vi "svx_Colormap Exec Commands.vi"(5 "Container ref":refnum<vi>, 6 "This VI":refnum<vi>, 7 "Colormap ref":refnum<vi>, 9 "Events":T2[](array[typedef])=[enum."[Data] Update"], 10 "State in":T1={"RefQueue"=refnum, "Properties/Undo"=refnum, "Bound"={"Width"=0, "Height"=0}, "Plot Area:Colors"={"FG Color"=11776947, "BG Color"=0}, "scale legend visible?"=FALSE, "graph palette visible?"=FALSE, "cursor palette visible?"=FALSE, "Ignore Array"=TRUE, "Smooth Update"=FALSE, "Z Scale"={"Z Scale.Scale Fit"=2, "Z Scale.Name Label.Text"="Amplitude", "Z Scale.Interpolate Color"=TRUE, "Visible"=TRUE, "Label Visible"=TRUE, "format string"="%#.2g", "Z Scale.Range"={"Minimum"=0.0, "Maximum"=500.0}}, "X Scale"={"X Scale.Scale Fit"=2, "X Scale.Offset and Multiplier"={"Offset"=0.0, "Multiplier"=1.0}, "X Scale.Name Label.Text"="Time", "X Scale.Range"={"Minimum"=0.0, "Maximum"=10.0}, "Visible"=TRUE, "Label Visible"=TRUE, "format string"="%#.2g"}, "Y Scale"={"Y Scale.Scale Fit"=2, "Y Scale.Offset and Multiplier"={"Offset"=0.0, "Multiplier"=1.0}, "Y Scale.Name Label.Text"="Frequency", "Y Scale.Range"={"Minimum"=0.0, "Maximum"=500.0}, "Visible"=TRUE, "Label Visible"=TRUE, "format string"="%#.2g"}, "Annotation List"=[], "Cursor List"=[], "Display Frequency Lines"=TRUE, "Display Order Lines"=TRUE, "Display Order text"=TRUE, "Display Frequency text"=TRUE, "Order Lineproperty"={"Line"={"Width"=1, "Style"=enum."Dash"}, "color"=0}, "Order Textproperty"={"Test size"=11, "color"=16777222, "background"=16777216}, "Orders"=[], "Frequency"=[], "Frequency Lineproperty"={"Line"={"Width"=1, "Style"=enum."Dash"}, "color"=0}, "Frequency Textproperty"={"Test size"=11, "color"=16777222, "background"=16777216}, "Display Order from Cursor"=FALSE, "Display Freq from Cursor"=FALSE, "Active Cursor"=0, "Selected Cursors"=[], "Cursor Move"=refnum, "Scale Range Change"=refnum}, 11 "Data in":T3 {"Y scale"."multiplier" format="%.2f"; "Y scale"."offset" format="%.2f"; "X scale"."multiplier" format="%.2f"; "X scale"."offset" format="%.2f"; "spectral map" format="%.2f"}) -> (2 "State out":T1={"RefQueue"=refnum, "Properties/Undo"=refnum, "Bound"={"Width"=0, "Height"=0}, "Plot Area:Colors"={"FG Color"=11776947, "BG Color"=0}, "scale legend visible?"=FALSE, "graph palette visible?"=FALSE, "cursor palette visible?"=FALSE, "Ignore Array"=TRUE, "Smooth Update"=FALSE, "Z Scale"={"Z Scale.Scale Fit"=2, "Z Scale.Name Label.Text"="Amplitude", "Z Scale.Interpolate Color"=TRUE, "Visible"=TRUE, "Label Visible"=TRUE, "format string"="%#.2g", "Z Scale.Range"={"Minimum"=0.0, "Maximum"=500.0}}, "X Scale"={"X Scale.Scale Fit"=2, "X Scale.Offset and Multiplier"={"Offset"=0.0, "Multiplier"=1.0}, "X Scale.Name Label.Text"="Time", "X Scale.Range"={"Minimum"=0.0, "Maximum"=10.0}, "Visible"=TRUE, "Label Visible"=TRUE, "format string"="%#.2g"}, "Y Scale"={"Y Scale.Scale Fit"=2, "Y Scale.Offset and Multiplier"={"Offset"=0.0, "Multiplier"=1.0}, "Y Scale.Name Label.Text"="Frequency", "Y Scale.Range"={"Minimum"=0.0, "Maximum"=500.0}, "Visible"=TRUE, "Label Visible"=TRUE, "format string"="%#.2g"}, "Annotation List"=[], "Cursor List"=[], "Display Frequency Lines"=TRUE, "Display Order Lines"=TRUE, "Display Order text"=TRUE, "Display Frequency text"=TRUE, "Order Lineproperty"={"Line"={"Width"=1, "Style"=enum."Dash"}, "color"=0}, "Order Textproperty"={"Test size"=11, "color"=16777222, "background"=16777216}, "Orders"=[], "Frequency"=[], "Frequency Lineproperty"={"Line"={"Width"=1, "Style"=enum."Dash"}, "color"=0}, "Frequency Textproperty"={"Test size"=11, "color"=16777222, "background"=16777216}, "Display Order from Cursor"=FALSE, "Display Freq from Cursor"=FALSE, "Active Cursor"=0, "Selected Cursors"=[], "Cursor Move"=refnum, "Scale Range Change"=refnum})   [LabVIEW 2017, in "SVX Colormap.xctl"]
uses:
  <vilib>/addons/_XControls/Colormap/SVX Colormap.xctl
  <vilib>/addons/_XControls/Colormap/subVIs/svx_Colormap Data.ctl
  <vilib>/addons/_XControls/Colormap/TypeDef/svx_Colormap_Event.ctl
  <vilib>/addons/_XControls/Colormap/subVIs/svx_Colormap State.ctl
  <vilib>/addons/_XControls/Colormap/TypeDef/svx_Colormap_InnerState.ctl
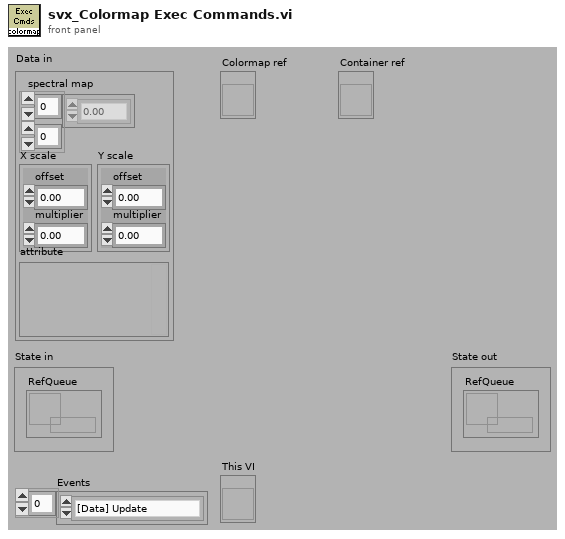
[diagram p1: front panel]
types:
  T1 = typedef "SVX Colormap.xctl/svx_Colormap State.ctl" = cluster{"RefQueue":refnum<queue>, "Properties/Undo":refnum<queue>, "Bound":cluster{"Width":u32, "Height":u32}, "Plot Area:Colors":cluster{"FG Color":u32, "BG Color":u32}, "scale legend visible?":bool, "graph palette visible?":bool, "cursor palette visible?":bool, "Ignore Array":bool, "Smooth Update":bool, "Z Scale":cluster{"Z Scale.Scale Fit":u8, "Z Scale.Name Label.Text":string, "Z Scale.Interpolate Color":bool, "Visible":bool, "Label Visible":bool, "format string":string, "Z Scale.Range":cluster{"Minimum":dbl, "Maximum":dbl}}, "X Scale":cluster{"X Scale.Scale Fit":u8, "X Scale.Offset and Multiplier":cluster{"Offset":dbl, "Multiplier":dbl}, "X Scale.Name Label.Text":string, "X Scale.Range":cluster{"Minimum":dbl, "Maximum":dbl}, "Visible":bool, "Label Visible":bool, "format string":string}, "Y Scale":cluster{"Y Scale.Scale Fit":u8, "Y Scale.Offset and Multiplier":cluster{"Offset":dbl, "Multiplier":dbl}, "Y Scale.Name Label.Text":string, "Y Scale.Range":cluster{"Minimum":dbl, "Maximum":dbl}, "Visible":bool, "Label Visible":bool, "format string":string}, "Annotation List":cluster{"Name":string, "Color":u32, "Style":u8, "Point Style":u8, "Name Visible":bool, "Allow Drag":bool, "Annotation Mode":u32, "Plot":i32, "Index":i32, "Position":cluster{"X":dbl, "Y":dbl}, "X Scale":u32, "Y Scale":u32, "Show Arrow":bool, "Lock Name":bool, "Plot Area":i32, "Label Offset":cluster{"X":dbl, "Y":dbl}}[], "Cursor List":cluster{"Name":string, "Color":u32, "Style":u8, "Point Style":u8, "Name Visible":bool, "Allow Drag":bool, "Cursor Mode":u32, "Plot":i32, "Index":i32, "Position":cluster{"X":dbl, "Y":dbl}, "X Scale":u32, "Y Scale":u32, "Watch Plots":i32[], "Watch All Plots":bool, "Plot Area":i32, "Label Offset":cluster{"X":dbl, "Y":dbl}}[], "Display Frequency Lines":bool, "Display Order Lines":bool, "Display Order text":bool, "Display Frequency text":bool, "Order Lineproperty":cluster{"Line":cluster{"Width":u16, "Style":enum32{"Solid", "Dash", "Dot", "DashDot", "DashDotDot"}}, "color":u32}, "Order Textproperty":cluster{"Test size":i16, "color":u32, "background":u32}, "Orders":dbl[], "Frequency":dbl[], "Frequency Lineproperty":cluster{"Line":cluster{"Width":u16, "Style":enum32{"Solid", "Dash", "Dot", "DashDot", "DashDotDot"}}, "color":u32}, "Frequency Textproperty":cluster{"Test size":i16, "color":u32, "background":u32}, "Display Order from Cursor":bool, "Display Freq from Cursor":bool, "Active Cursor":u32, "Selected Cursors":u32[], "Cursor Move":refnum<user-event>, "Scale Range Change":refnum<user-event>}
  T2 = typedef "SVX Colormap.xctl/svx_Colormap_Event.ctl" = enum16{"None", "[Axis] X Range", "[Axis] Y Range", "[Axis] Z Range", "[Axis] Range", "[Axis] X FString", "[Axis] Y FString", "[Axis] Z FString", "[Axis] X Name", "[Axis] X ScaleVis", "[Axis] X NameVis", "[Axis] Y Name", "[Axis] Y ScaleVis", "[Axis] Y NameVis", "[Axis] Z Name", "[Axis] Z ScaleVis", "[Axis] Z NameVis", "[Image] Line", "[Axis] Z Interp", "[Data] Update", "[Layout] Resize", "[ColorTable] Ignore Array", "[Legend] ScaleVis", "[Legend] GPVis", "[Legend] CPVis", "[Smooth] Update", "[Cursor] Update", "[Plot Area] Colors", "[Size] Minimum", "[Annotation] Update", "[Properties Dialog]", "[Axis] Autoscale X", "[Axis] Autoscale Y", "[Axis] Autoscale Z"}
  T3 = typedef "SVX Colormap.xctl/svx_Colormap Data.ctl" = cluster{"spectral map":dbl[][], "X scale":cluster{"offset":dbl, "multiplier":dbl}, "Y scale":cluster{"offset":dbl, "multiplier":dbl}, "attribute":variant}
  T4 = cluster{"Name":string, "Color":u32, "Style":u8, "Point Style":u8, "Name Visible":bool, "Allow Drag":bool, "Cursor Mode":u32, "Plot":i32, "Index":i32, "Position":cluster{"X":dbl, "Y":dbl}, "X Scale":u32, "Y Scale":u32, "Watch Plots":i32[], "Watch All Plots":bool, "Plot Area":i32, "Label Offset":cluster{"X":dbl, "Y":dbl}}[]
  T5 = cluster{"Name":string, "Color":u32, "Style":u8, "Point Style":u8, "Name Visible":bool, "Allow Drag":bool, "Annotation Mode":u32, "Plot":i32, "Index":i32, "Position":cluster{"X":dbl, "Y":dbl}, "X Scale":u32, "Y Scale":u32, "Show Arrow":bool, "Lock Name":bool, "Plot Area":i32, "Label Offset":cluster{"X":dbl, "Y":dbl}}[]
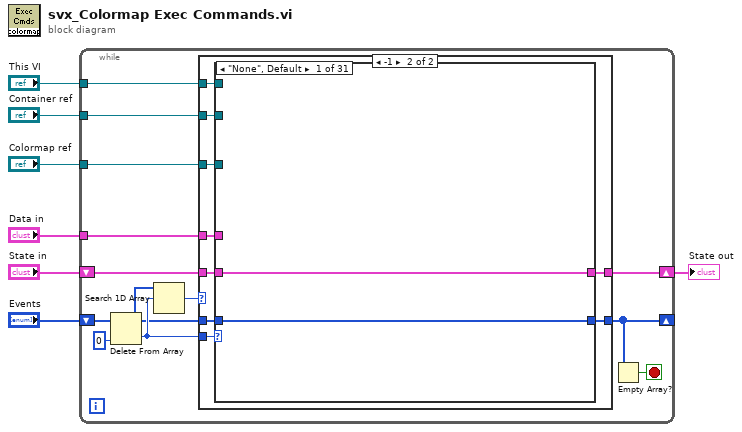
[diagram p0: block diagram]
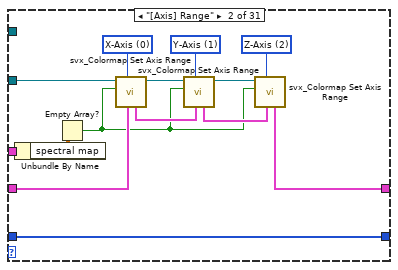
[diagram p3: hidden frame]
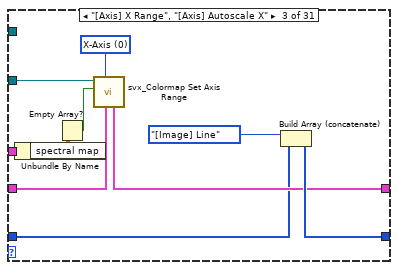
[diagram p4: hidden frame]
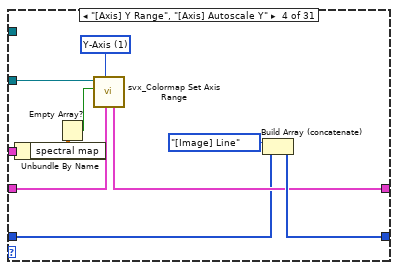
[diagram p5: hidden frame]
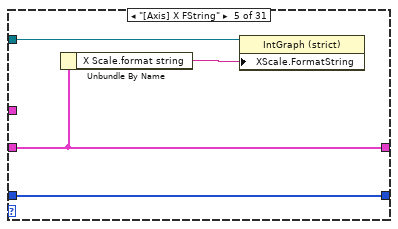
[diagram p6: hidden frame]
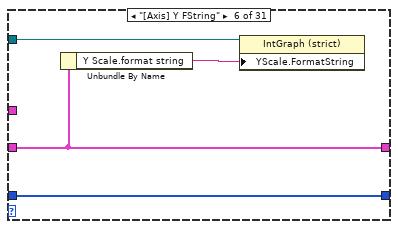
[diagram p7: hidden frame]
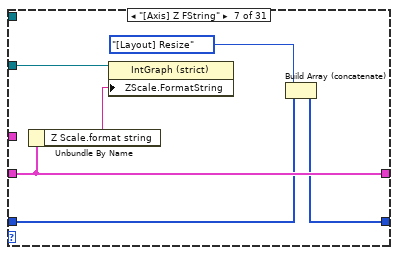
[diagram p8: hidden frame]
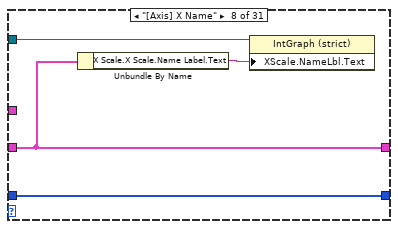
[diagram p9: hidden frame]
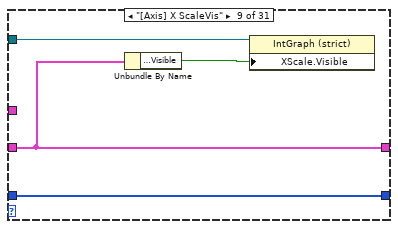
[diagram p10: hidden frame]
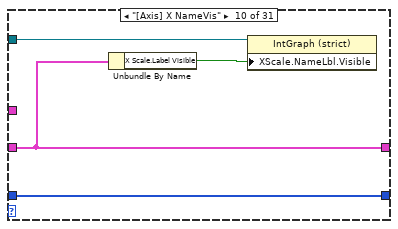
[diagram p11: hidden frame]
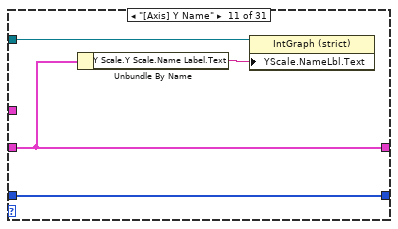
[diagram p12: hidden frame]
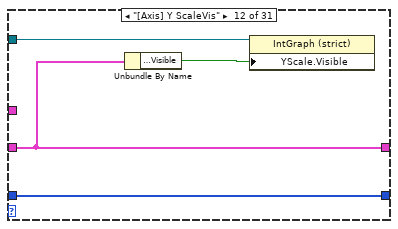
[diagram p13: hidden frame]
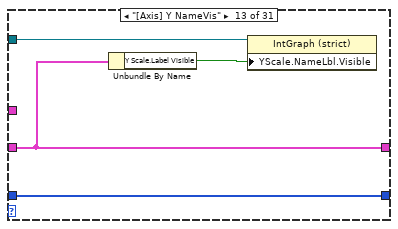
[diagram p14: hidden frame]
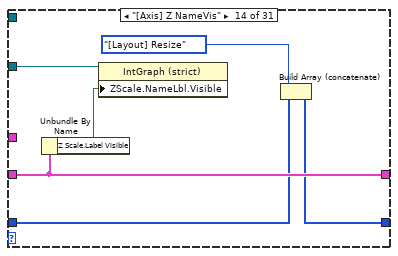
[diagram p15: hidden frame]
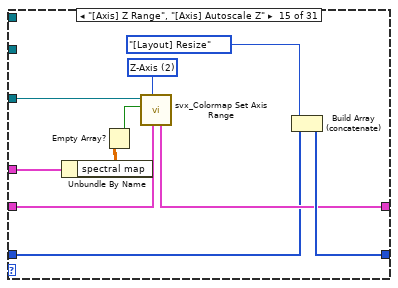
[diagram p16: hidden frame]
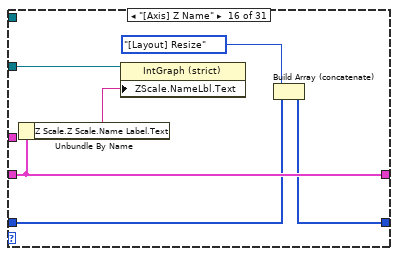
[diagram p17: hidden frame]
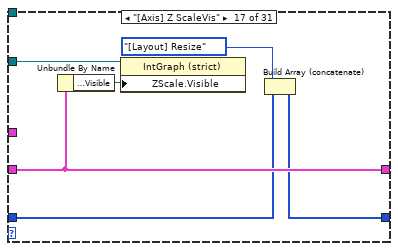
[diagram p18: hidden frame]
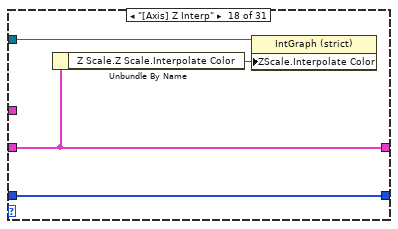
[diagram p19: hidden frame]
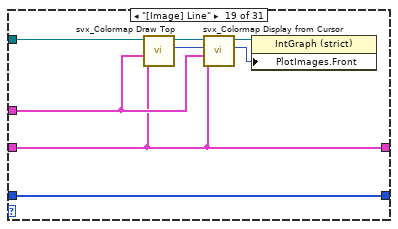
[diagram p20: hidden frame]
diagram:
  n1 = while {
    tunnel: "Data in" -> [w20]
    tunnel: "Colormap ref" -> [w19]
    shift-right: [w13] -> w1
    shift-left: "State in" -> [w18]
    shift-right: [w15] -> _
    shift-left: "Events" -> [w16]
    tunnel: "Container ref" -> [w12]
    tunnel: "This VI" -> [w8]
    stop <- w14 stop-if-true
    n2 = Delete From Array(array=w16, index=0) -> (deleted portion=w11:T2, array with subset deleted=w10:T2[])  [unwired: 1 in]
    n3 = Search 1D Array(1D array=w10, element=w11) -> (index of element=w9:i32)  [unwired: 1 in]
    n4 = case shown="-1" w9 {
      tunnel: w20 -> [_ w31]
      tunnel: w19 -> [_ w30]
      tunnel: w18 -> [w22 w29]
      tunnel: [w21 w28] -> w15
      tunnel: [w22 w27] -> w13
      tunnel: w12 -> [_ w26]
      tunnel: w11 -> [_ w25]
      tunnel: w10 -> [w21 w24]
      tunnel: w8 -> [_ w23]
      frame Default {
      }
      frame -1 {
        n5 = case shown="\"None\", Default" w25 {
          tunnel: w31 -> [_ w45 w55 w65 _ _ _ _ _ _ _ _ _ _ w116 _ _ _ w144 _ w155 _ _ _ _ _ _ _ _ _ _]
          tunnel: w29 -> [w33 w43 w53 w63 w69 w73 w80 w84 w88 w92 w96 w100 w104 w111 w115 w126 w133 w135 w138 w147 w154 w162 w172 w178 w185 w189 w202 w206 w213 w218 w223]
          tunnel: w30 -> [_ w46 w56 w66 w71 w75 w78 w85 w89 w93 w97 w101 w105 w108 w118 w124 w130 w137 w145 w148 w156 w167 w174 w180 w187 w191 w204 w208 _ w221 _]
          tunnel: w24 -> [w32 w34 w48 w59 w68 w72 w77 w83 w87 w91 w95 w99 w103 w106 w113 w122 w128 w134 w143 w146 w152 w161 w169 w175 w182 w188 w199 w205 w212 w219 _]
          tunnel: [w32 w34 w51 w61 w68 w72 w79 w83 w87 w91 w95 w99 w103 w110 w121 w125 w132 w134 w143 w146 w151 w161 w171 w177 w184 w188 w198 w205 w212 w219 w222] -> w28
          tunnel: [w33 w35 w50 w60 w69 w73 w80 w84 w88 w92 w96 w100 w104 w111 w114 w126 w133 w135 w138 w147 w153 w162 w172 w178 w185 w189 w202 w206 w213 w218 w223] -> w27
          tunnel: w26 -> [_ _ _ _ _ _ _ _ _ _ _ _ _ _ _ _ _ _ _ w149 _ _ _ _ _ _ _ _ _ _ _]
          tunnel: w23 -> [_ _ _ _ _ _ _ _ _ _ _ _ _ _ _ _ _ _ _ _ _ _ _ _ _ _ _ _ w214 _ _]
          frame "None", Default {
          }
          frame "[Axis] Range" {
            w41 = u16 2 items=["X-Axis", "Y-Axis", "Z-Axis"] ("axis selection")
            w42 = u16 1 items=["X-Axis", "Y-Axis", "Z-Axis"] ("axis selection")
            w47 = u16 0 items=["X-Axis", "Y-Axis", "Z-Axis"] ("axis selection")
            n6 = Unbundle By Name(w45) -> ("spectral map"=w44:dbl[][])
            n7 = Empty Array?(array=w44) -> (empty?=w36:bool)
            n8 = call <vilib>:"svx_Colormap Set Axis Range.vi"("State in"=w43, "axis selection"=w47, "empty?"=w36, "Color Map in"=w46) -> ("Color Map out"=w39:refnum<vi>, "State out"=w40:T1)  [unwired: 5 in, 1 out]
            n9 = call <vilib>:"svx_Colormap Set Axis Range.vi"("State in"=w40, "axis selection"=w42, "empty?"=w36, "Color Map in"=w39) -> ("Color Map out"=w37:refnum<vi>, "State out"=w38:T1)  [unwired: 5 in, 1 out]
            n10 = call <vilib>:"svx_Colormap Set Axis Range.vi"("State in"=w38, "axis selection"=w41, "empty?"=w36, "Color Map in"=w37) -> ("State out"=w35:T1)  [unwired: 5 in, 2 out]
          }
          frame "[Axis] X Range", "[Axis] Autoscale X" {
            w57 = u16 0 items=["X-Axis", "Y-Axis", "Z-Axis"] ("axis selection")
            n11 = Unbundle By Name(w55) -> ("spectral map"=w54:dbl[][])
            n12 = Empty Array?(array=w54) -> (empty?=w52:bool)
            n13 = call <vilib>:"svx_Colormap Set Axis Range.vi"("State in"=w53, "axis selection"=w57, "empty?"=w52, "Color Map in"=w56) -> ("State out"=w50:T1)  [unwired: 5 in, 2 out]
            n14 = Build Array (concatenate)(svx_Colormap_Event."[Image] Line" ("Property Page User Events"), w48) -> (w51:T2[])
          }
          frame "[Axis] Y Range", "[Axis] Autoscale Y" {
            w67 = u16 1 items=["X-Axis", "Y-Axis", "Z-Axis"] ("axis selection")
            n15 = Unbundle By Name(w65) -> ("spectral map"=w64:dbl[][])
            n16 = Empty Array?(array=w64) -> (empty?=w62:bool)
            n17 = call <vilib>:"svx_Colormap Set Axis Range.vi"("State in"=w63, "axis selection"=w67, "empty?"=w62, "Color Map in"=w66) -> ("State out"=w60:T1)  [unwired: 5 in, 2 out]
            n18 = Build Array (concatenate)(svx_Colormap_Event."[Image] Line" ("Property Page User Events"), w59) -> (w61:T2[])
          }
          frame "[Axis] X FString" {
            n19 = Unbundle By Name(w69) -> ("X Scale.format string"=w70:string)
            n20 = property class="IntGraph (strict)"(reference=w71, "XScale.FormatString"=w70) -> ()  [unwired: 1 in, 2 out]
          }
          frame "[Axis] Y FString" {
            n21 = Unbundle By Name(w73) -> ("Y Scale.format string"=w74:string)
            n22 = property class="IntGraph (strict)"(reference=w75, "YScale.FormatString"=w74) -> ()  [unwired: 1 in, 2 out]
          }
          frame "[Axis] Z FString" {
            n23 = Unbundle By Name(w80) -> ("Z Scale.format string"=w81:string)
            n24 = property class="IntGraph (strict)"(reference=w78, "ZScale.FormatString"=w81) -> ()  [unwired: 1 in, 2 out]
            n25 = Build Array (concatenate)(svx_Colormap_Event."[Layout] Resize" ("Property Page User Events"), w77) -> (w79:T2[])
          }
          frame "[Axis] X Name" {
            n26 = Unbundle By Name(w84) -> ("X Scale.X Scale.Name Label.Text"=w82:string)
            n27 = property class="IntGraph (strict)"(reference=w85, "XScale.NameLbl.Text"=w82) -> ()  [unwired: 1 in, 2 out]
          }
          frame "[Axis] X ScaleVis" {
            n28 = Unbundle By Name(w88) -> ("X Scale.Visible"=w86:bool)
            n29 = property class="IntGraph (strict)"(reference=w89, "XScale.Visible"=w86) -> ()  [unwired: 1 in, 2 out]
          }
          frame "[Axis] X NameVis" {
            n30 = Unbundle By Name(w92) -> ("X Scale.Label Visible"=w90:bool)
            n31 = property class="IntGraph (strict)"(reference=w93, "XScale.NameLbl.Visible"=w90) -> ()  [unwired: 1 in, 2 out]
          }
          frame "[Axis] Y Name" {
            n32 = Unbundle By Name(w96) -> ("Y Scale.Y Scale.Name Label.Text"=w94:string)
            n33 = property class="IntGraph (strict)"(reference=w97, "YScale.NameLbl.Text"=w94) -> ()  [unwired: 1 in, 2 out]
          }
          frame "[Axis] Y ScaleVis" {
            n34 = Unbundle By Name(w100) -> ("Y Scale.Visible"=w98:bool)
            n35 = property class="IntGraph (strict)"(reference=w101, "YScale.Visible"=w98) -> ()  [unwired: 1 in, 2 out]
          }
          frame "[Axis] Y NameVis" {
            n36 = Unbundle By Name(w104) -> ("Y Scale.Label Visible"=w102:bool)
            n37 = property class="IntGraph (strict)"(reference=w105, "YScale.NameLbl.Visible"=w102) -> ()  [unwired: 1 in, 2 out]
          }
          frame "[Axis] Z NameVis" {
            n38 = Unbundle By Name(w111) -> ("Z Scale.Label Visible"=w109:bool)
            n39 = property class="IntGraph (strict)"(reference=w108, "ZScale.NameLbl.Visible"=w109) -> ()  [unwired: 1 in, 2 out]
            n40 = Build Array (concatenate)(svx_Colormap_Event."[Layout] Resize" ("Property Page User Events"), w106) -> (w110:T2[])
          }
          frame "[Axis] Z Range", "[Axis] Autoscale Z" {
            w117 = u16 2 items=["X-Axis", "Y-Axis", "Z-Axis"] ("axis selection")
            n41 = Unbundle By Name(w116) -> ("spectral map"=w120:dbl[][])
            n42 = Empty Array?(array=w120) -> (empty?=w119:bool)
            n43 = call <vilib>:"svx_Colormap Set Axis Range.vi"("State in"=w115, "axis selection"=w117, "empty?"=w119, "Color Map in"=w118) -> ("State out"=w114:T1)  [unwired: 5 in, 2 out]
            n44 = Build Array (concatenate)(svx_Colormap_Event."[Layout] Resize" ("Property Page User Events"), w113) -> (w121:T2[])
          }
          frame "[Axis] Z Name" {
            n45 = Unbundle By Name(w126) -> ("Z Scale.Z Scale.Name Label.Text"=w127:string)
            n46 = property class="IntGraph (strict)"(reference=w124, "ZScale.NameLbl.Text"=w127) -> ()  [unwired: 1 in, 2 out]
            n47 = Build Array (concatenate)(svx_Colormap_Event."[Layout] Resize" ("Property Page User Events"), w122) -> (w125:T2[])
          }
          frame "[Axis] Z ScaleVis" {
            n48 = Unbundle By Name(w133) -> ("Z Scale.Visible"=w131:bool)
            n49 = property class="IntGraph (strict)"(reference=w130, "ZScale.Visible"=w131) -> ()  [unwired: 1 in, 2 out]
            n50 = Build Array (concatenate)(svx_Colormap_Event."[Layout] Resize" ("Property Page User Events"), w128) -> (w132:T2[])
          }
          frame "[Axis] Z Interp" {
            n51 = Unbundle By Name(w135) -> ("Z Scale.Z Scale.Interpolate Color"=w136:bool)
            n52 = property class="IntGraph (strict)"(reference=w137, "ZScale.Interpolate Color"=w136) -> ()  [unwired: 1 in, 2 out]
          }
          frame "[Image] Line" {
            n53 = call <vilib>:"svx_Colormap Draw Top.vi"("State"=w138, "Data In"=w144, "Color Map in"=w145) -> ("new picture out"=w142:picture, "Color Map out"=w141:refnum<vi>)  [unwired: 7 in]
            n54 = call <vilib>:"svx_Colormap Display from Cursor.vi"("State"=w138, "Data In"=w144, "new picture in"=w142, "Color Map in"=w141) -> ("new picture out"=w139:picture, "Color Map out"=w140:refnum<vi>)  [unwired: 6 in]
            n55 = property class="IntGraph (strict)"(reference=w140, "PlotImages.Front"=w139) -> ()  [unwired: 1 in, 2 out]
          }
          frame "[Layout] Resize" {
            n56 = call <vilib>:"svx_Colormap Resize Pane for Scale and Cursor Legend.vi"("Color Map in"=w148, "Container ref"=w149) -> ()  [unwired: 10 in]
          }
          frame "[Data] Update" {
            w150 = T2[] [enum."[ColorTable] Ignore Array", enum."[Axis] Range", enum."[Image] Line"] items=["None", "[Axis] X Range", "[Axis] Y Range", "[Axis] Z Range", "[Axis] Range", "[Axis] X FString", "[Axis] Y FString", "[Axis] Z FString", "[Axis] X Name", "[Axis] X ScaleVis", "[Axis] X NameVis", "[Axis] Y Name", "[Axis] Y ScaleVis", "[Axis] Y NameVis", "[Axis] Z Name", "[Axis] Z ScaleVis", "[Axis] Z NameVis", "[Image] Line", "[Axis] Z Interp", "[Data] Update", "[Layout] Resize", "[ColorTable] Ignore Array", "[Legend] ScaleVis", "[Legend] GPVis", "[Legend] CPVis", "[Smooth] Update", "[Cursor] Update", "[Plot Area] Colors", "[Size] Minimum", "[Annotation] Update", "[Properties Dialog]", "[Axis] Autoscale X", "[Axis] Autoscale Y", "[Axis] Autoscale Z"]
            n57 = Unbundle By Name(w155) -> ("X scale"=w159:cluster{"offset":dbl, "multiplier":dbl}, "Y scale"=w158:cluster{"offset":dbl, "multiplier":dbl}, "spectral map"=w157:dbl[][])
            n58 = property class="IntGraph (strict)"(reference=w156, "XScale.Ofst&Mult"=w159, "YScale.Ofst&Mult"=w158, "Val(Sgnl)"=w157) -> ()  [unwired: 1 in, 2 out]
            n59 = Bundle By Name(cluster=w154, "X Scale.X Scale.Offset and Multiplier"=w159, "Y Scale.Y Scale.Offset and Multiplier"=w158) -> (w153:T1)
            n60 = Build Array (concatenate)(w150, w152) -> (w151:T2[])
          }
          frame "[ColorTable] Ignore Array" {
            w165 = u32[] [0, 0, 2, 4, 6, 8, 10, 12, 14, 16, 18, 20, 22, 24, 26, 28, 30, 32, 34, 36, 38, 40, 42, 44, 46, 48, 50, 52, 54, 56, 58, 60, 62, 64, 66, 68, 70, 72, 74, 76, 78, 80, 82, 84, 86, 88, 90, 92, 94, 96, 98, 100, 102, 104, 106, 108, 110, 112, 114, 116, 118, 120, 122, 124, 126, 128, 130, 132, 134, 136, 138, 140, 142, 144, 146, 148, 150, 152, 154, 156, 158, 160, 162, 164, 166, 168, 170, 172, 174, 176, 178, 180, 182, 184, 186, 188, 190, 192, 194, 196, 198, 200, 202, 204, 206, 208, 210, 212, 214, 216, 218, 220, 222, 224, 226, 228, 230, 232, 234, 236, 238, 240, 242, 244, 246, 248, 250, 252, 255, 131839, 263423, 395007, 526591, 658175, 789759, 921343, 1052927, 1184511, 1316095, 1447679, 1579263, 1710847, 1842431, 1974015, 2105599, 2237183, 2368767, 2500351, 2631935, 2763519, 2895103, 3026687, 3158271, 3289855, 3421439, 3553023, 3684607, 3816191, 3947775, 4079359, 4210943, 4342527, 4474111, 4605695, 4737279, 4868863, 5000447, 5132031, 5263615, 5395199, 5526783, 5658367, 5789951, 5921535, 6053119, 6184703, 6316287, 6447871, 6579455, 6711039, 6842623, 6974207, 7105791, 7237375, 7368959, 7500543, 7632127, 7763711, 7895295, 8026879, 8158463, 8290047, 8421631, 8553215, 8684799, 8816383, 8947967, 9079551, 9211135, 9342719, 9474303, 9605887, 9737471, 9869055, 10000639, 10132223, 10263807, 10395391, 10526975, 10658559, 10790143, 10921727, 11053311, 11184895, 11316479, 11448063, 11579647, 11711231, 11842815, 11974399, 12105983, 12237567, 12369151, 12500735, 12632319, 12763903, 12895487, 13027071, 13158655, 13290239, 13421823, 13553407, 13684991, 13816575, 13948159, 14079743, 14211327, 14342911, 14474495, 14606079, 14737663, 14869247, 15000831, 15132415, 15263999, 15395583, 15527167, 15658751, 15790335, 15921919, 16053503, 16185087, 16316671, 16448255, 16579839, 16777215]  # Color Table
            w166 = u32[] [0, 8388863, 8257791, 8061183, 7930111, 7733503, 7602431, 7405823, 7274751, 7078143, 6947071, 6750463, 6619391, 6422783, 6291711, 6095103, 5964031, 5767423, 5636351, 5439743, 5308671, 5112063, 4980991, 4784383, 4653311, 4456703, 4325631, 4129023, 3932415, 3801343, 3604735, 3473663, 3277055, 3145983, 2949375, 2818303, 2621695, 2490623, 2294015, 2162943, 1966335, 1835263, 1638655, 1507583, 1310975, 1179903, 983295, 852223, 655615, 524543, 327935, 196863, 511, 1791, 3071, 4351, 5631, 6911, 8191, 9471, 10751, 12031, 13311, 14591, 15871, 17151, 18431, 19711, 20991, 22271, 23551, 24831, 26111, 27391, 28671, 29951, 31231, 32511, 33791, 35071, 36351, 37631, 38911, 40191, 41471, 42751, 44031, 45311, 46591, 47871, 49151, 50431, 51711, 52991, 54271, 55551, 56831, 58111, 59391, 60671, 61951, 63231, 64511, 65532, 65527, 65522, 65517, 65512, 65507, 65502, 65497, 65492, 65487, 65482, 65477, 65472, 65467, 65462, 65457, 65452, 65447, 65442, 65437, 65432, 65427, 65422, 65417, 65412, 65407, 65402, 65397, 65392, 65387, 65382, 65377, 65372, 65367, 65362, 65357, 65352, 65347, 65342, 65337, 65332, 65327, 65322, 65317, 65312, 65307, 65302, 65297, 65292, 65287, 65282, 261888, 589568, 917248, 1244928, 1572608, 1900288, 2227968, 2555648, 2883328, 3211008, 3538688, 3866368, 4194048, 4521728, 4849408, 5177088, 5504768, 5832448, 6160128, 6487808, 6815488, 7143168, 7470848, 7798528, 8126208, 8453888, 8781568, 9109248, 9436928, 9764608, 10092288, 10419968, 10747648, 11075328, 11403008, 11730688, 12058368, 12386048, 12713728, 13041408, 13369088, 13696768, 14024448, 14352128, 14679808, 15007488, 15335168, 15662848, 15990528, 16318208, 16645888, 16775936, 16774656, 16773376, 16772096, 16770816, 16769536, 16768256, 16766976, 16765696, 16764416, 16763136, 16761856, 16760576, 16759296, 16758016, 16756736, 16755456, 16754176, 16752896, 16751616, 16750336, 16749056, 16747776, 16746496, 16745216, 16743936, 16742656, 16741376, 16740096, 16738816, 16737536, 16736256, 16734976, 16733696, 16732416, 16731136, 16729856, 16728576, 16727296, 16726016, 16724736, 16723456, 16722176, 16720896, 16719616, 16718336, 16717056, 16715776, 16714496, 16713216, 16711680]  # rainbow
            n61 = Unbundle By Name(w162) -> ("Ignore Array"=w164:bool)
            n62 = Select(t=w166, s=w164, f=w165) -> (s? t:f=w163:u32[])
            n63 = property class="IntGraph (strict)"(reference=w167, "Ignore Array"=TRUE, "Color Table"=w163) -> ()  [unwired: 1 in, 2 out]
          }
          frame "[Legend] ScaleVis" {
            n64 = Unbundle By Name(w172) -> ("scale legend visible?"=w173:bool)
            n65 = property class="IntGraph (strict)"(reference=w174, "ScaleLegendVis"=w173) -> ()  [unwired: 1 in, 2 out]
            n66 = Build Array (concatenate)(svx_Colormap_Event."[Size] Minimum" ("Property Page User Events"), svx_Colormap_Event."[Layout] Resize" ("Property Page User Events"), w169) -> (w171:T2[])
          }
          frame "[Legend] GPVis" {
            n67 = Unbundle By Name(w178) -> ("graph palette visible?"=w179:bool)
            n68 = property class="IntGraph (strict)"(reference=w180, "Palette Visible"=w179) -> ()  [unwired: 1 in, 2 out]
            n69 = Build Array (concatenate)(svx_Colormap_Event."[Layout] Resize" ("Property Page User Events"), w175) -> (w177:T2[])
          }
          frame "[Legend] CPVis" {
            n70 = Unbundle By Name(w185) -> ("cursor palette visible?"=w186:bool)
            n71 = property class="IntGraph (strict)"(reference=w187, "Cursor Palette Vis"=w186) -> ()  [unwired: 1 in, 2 out]
            n72 = Build Array (concatenate)(svx_Colormap_Event."[Size] Minimum" ("Property Page User Events"), svx_Colormap_Event."[Layout] Resize" ("Property Page User Events"), w182) -> (w184:T2[])
          }
          frame "[Smooth] Update" {
            n73 = Unbundle By Name(w189) -> ("Smooth Update"=w190:bool)
            n74 = property class="IntGraph (strict)"(reference=w191, "Smooth Update"=w190) -> ()  [unwired: 1 in, 2 out]
          }
          frame "[Cursor] Update" {
            w195 = T2[] [] items=["None", "[Axis] X Range", "[Axis] Y Range", "[Axis] Z Range", "[Axis] Range", "[Axis] X FString", "[Axis] Y FString", "[Axis] Z FString", "[Axis] X Name", "[Axis] X ScaleVis", "[Axis] X NameVis", "[Axis] Y Name", "[Axis] Y ScaleVis", "[Axis] Y NameVis", "[Axis] Z Name", "[Axis] Z ScaleVis", "[Axis] Z NameVis", "[Image] Line", "[Axis] Z Interp", "[Data] Update", "[Layout] Resize", "[ColorTable] Ignore Array", "[Legend] ScaleVis", "[Legend] GPVis", "[Legend] CPVis", "[Smooth] Update", "[Cursor] Update", "[Plot Area] Colors", "[Size] Minimum", "[Annotation] Update", "[Properties Dialog]", "[Axis] Autoscale X", "[Axis] Autoscale Y", "[Axis] Autoscale Z"] ("f")
            w196 = T2[] [enum."[Image] Line"] items=["None", "[Axis] X Range", "[Axis] Y Range", "[Axis] Z Range", "[Axis] Range", "[Axis] X FString", "[Axis] Y FString", "[Axis] Z FString", "[Axis] X Name", "[Axis] X ScaleVis", "[Axis] X NameVis", "[Axis] Y Name", "[Axis] Y ScaleVis", "[Axis] Y NameVis", "[Axis] Z Name", "[Axis] Z ScaleVis", "[Axis] Z NameVis", "[Image] Line", "[Axis] Z Interp", "[Data] Update", "[Layout] Resize", "[ColorTable] Ignore Array", "[Legend] ScaleVis", "[Legend] GPVis", "[Legend] CPVis", "[Smooth] Update", "[Cursor] Update", "[Plot Area] Colors", "[Size] Minimum", "[Annotation] Update", "[Properties Dialog]", "[Axis] Autoscale X", "[Axis] Autoscale Y", "[Axis] Autoscale Z"] ("array")
            n75 = Unbundle By Name(w202) -> ("Cursor List"=w203:T4, "Selected Cursors"=w193:u32[], "Display Order from Cursor"=w201:bool, "Display Freq from Cursor"=w200:bool)
            n76 = property class="IntGraph (strict)"(reference=w204, "CrsrLis"=w203) -> (reference out=w192:refnum<vi>)  [unwired: 1 in, 1 out]
            n77 = Or(x=w201, y=w200) -> (x .or. y?=w197:bool)
            n78 = Select(t=w196, s=w197, f=w195) -> (s? t:f=w194:T2[])
            n79 = property class="IntGraph (strict)"(reference=w192, "Selected Cursors"=w193) -> ()  [unwired: 1 in, 2 out]
            n80 = Build Array (concatenate)(w194, w199) -> (w198:T2[])
          }
          frame "[Plot Area] Colors" {
            n81 = Unbundle By Name(w206) -> ("Plot Area:Colors"=w207:cluster{"FG Color":u32, "BG Color":u32})
            n82 = property class="IntGraph (strict)"(reference=w208, "Plot Area Colors"=w207) -> ()  [unwired: 1 in, 2 out]
          }
          frame "[Size] Minimum" {
            n83 = Unbundle By Name(w213) -> ("scale legend visible?"=w211:bool, "cursor palette visible?"=w210:bool)
            n84 = Or(x=w211, y=w210) -> (x .or. y?=w209:bool)
            n85 = Select(t=cluster{"Horizontal":i16, "Vertical":i16} {"Horizontal"=350, "Vertical"=250} ("Front Panel Window:Minimum Size"), s=w209, f=cluster{"Horizontal":i16, "Vertical":i16} {"Horizontal"=350, "Vertical"=150}) -> (s? t:f=w215:cluster{"Horizontal":i16, "Vertical":i16})
            n86 = property class="FcdVI"(reference=w214, "Minimum Panel Size"=w215) -> ()  [unwired: 1 in, 2 out]
          }
          frame "[Annotation] Update" {
            n87 = Unbundle By Name(w218) -> ("Annotation List"=w220:T5)
            n88 = property class="IntGraph (strict)"(reference=w221, "AnntList"=w220) -> ()  [unwired: 1 in, 2 out]
          }
          frame "[Properties Dialog]" {
            w222 = T2[] [enum."[Axis] Range", enum."[Axis] X FString", enum."[Axis] Y FString", enum."[Axis] Z FString", enum."[Axis] X Name", enum."[Axis] X ScaleVis", enum."[Axis] X NameVis", enum."[Axis] Y Name", enum."[Axis] Y ScaleVis", enum."[Axis] Y NameVis", enum."[Axis] Z Name", enum."[Axis] Z ScaleVis", enum."[Axis] Z NameVis", enum."[Axis] Z Interp", enum."[ColorTable] Ignore Array", enum."[Smooth] Update", enum."[Image] Line"] items=["None", "[Axis] X Range", "[Axis] Y Range", "[Axis] Z Range", "[Axis] Range", "[Axis] X FString", "[Axis] Y FString", "[Axis] Z FString", "[Axis] X Name", "[Axis] X ScaleVis", "[Axis] X NameVis", "[Axis] Y Name", "[Axis] Y ScaleVis", "[Axis] Y NameVis", "[Axis] Z Name", "[Axis] Z ScaleVis", "[Axis] Z NameVis", "[Image] Line", "[Axis] Z Interp", "[Data] Update", "[Layout] Resize", "[ColorTable] Ignore Array", "[Legend] ScaleVis", "[Legend] GPVis", "[Legend] CPVis", "[Smooth] Update", "[Cursor] Update", "[Plot Area] Colors", "[Size] Minimum", "[Annotation] Update", "[Properties Dialog]", "[Axis] Autoscale X", "[Axis] Autoscale Y", "[Axis] Autoscale Z"] ("remaining elements")
          }
        }
      }
    }
    n89 = Empty Array?(array=w15) -> (empty?=w14:bool)
  }
  "State out" <- w1
